vi "Get ManagementBaseObj Props.vi"(3 ".NET Refnum in":refnum<k24>, 4 "error in":errorcluster, 6 "Property Names":string[](array[string])) -> (0 "dup .NET Refnum":refnum<k24>, 1 "error out":errorcluster, 5 "Property Values":string[](array[string]))   [LabVIEW 2016]
uses:
  System.Management
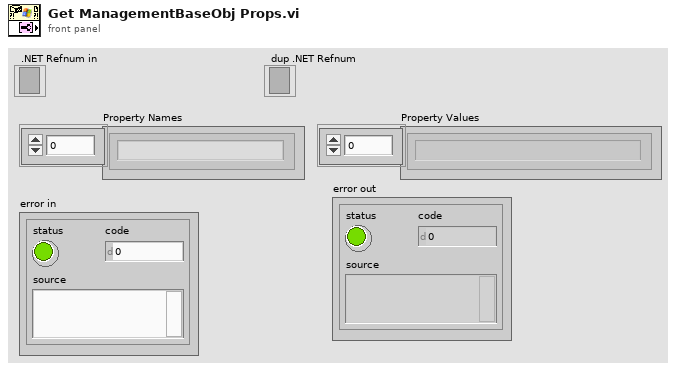
[diagram p1: front panel]
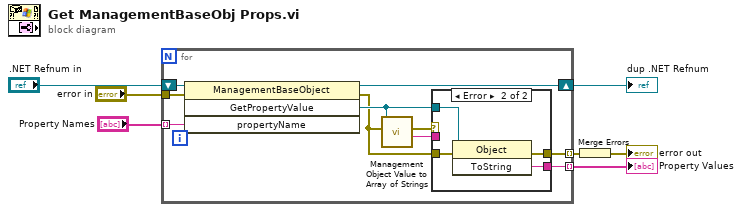
[diagram p0: block diagram]
diagram:
  n1 = for {
    tunnel: [w9] -> w7 mode=indexing
    tunnel: "error in" -> [w17]
    tunnel: [w8] -> w2 mode=indexing
    shift-right: [w14] -> w4
    shift-left: ".NET Refnum in" -> [w16]
    tunnel: "Property Names" -> [w15] mode=indexing
    n2 = invoke class="ManagementBaseObject" method="GetPropertyValue"(reference=w16, error in=w17, "propertyName"=w15) -> (reference out=w14:refnum<k24>, error out=w10:errorcluster, "GetPropertyValue"=w11:refnum<k24>)  [unwired: 1 in, 1 out]
    n3 = call "Management Object Value to Array of Strings.vi"(".NET Refnum in"=w11, "error in"=w10) -> ("error out"=w13:errorcluster, "Spreadsheet string"=w12:string)  [unwired: 4 in, 2 out]
    n4 = case shown="Error" w13 {
      selector: w13 -> [w19 _]
      tunnel: [w18 w23] -> w9
      tunnel: [w19 w22] -> w8
      tunnel: w11 -> [_ w21]
      tunnel: w10 -> [_ w20]
      tunnel: w12 -> [w18 _]
      frame No Error {
      }
      frame Error {
        n5 = invoke class="Object" method="ToString"(reference=w21, error in=w20) -> (error out=w22:errorcluster, "ToString"=w23:string)  [unwired: 1 in, 1 out]
      }
    }
  }
  "Property Values" <- w7
  "dup .NET Refnum" <- w4
  n6 = Merge Errors(w2) -> (→"error out":errorcluster)
